vi "Inbetriebnahme_Marc.vi"() -> ()   [LabVIEW 2016]
panel:
  in  "Wicklungszahl n2 theoretisch":dbl=700.0
  out "Neukurve":cluster{"Y":dbl[], "Y":dbl[]}[](graph) caption="XY-Graph"
  in  "lm [cm]":dbl=94.0
  in  "Querschnitt A":dbl=45.0
  in  "Faktor Runge Kutta":dbl=700.0
  in  "Wicklungszahl n1 theoretisch":dbl=700.0
  in  "ShuntWiderstand [Ohm]":dbl=1.0
  in  "maximale Spannung":dbl=10.0
  in  "Messpunkte Oszi (6000)":i32=6000
  in  "VISA Name OZ in(OZ)":refnum<visa-resource-name>="USB0::0x0957::0x179B::MY54313507::INSTR"
  out "error out":errorcluster
  in  "Frequenz [Hz]":dbl
  in  "Spannungs Abweichung":dbl
  in  "Error_in":errorcluster
  in  "VISA Name FG in(FG)":refnum<visa-resource-name>="USB0::0x0957::0x0407::MY44043889::INSTR"
  # "Parameter Frequenzgenerator und Oszi"
  # "Parameter Messuaufbau"
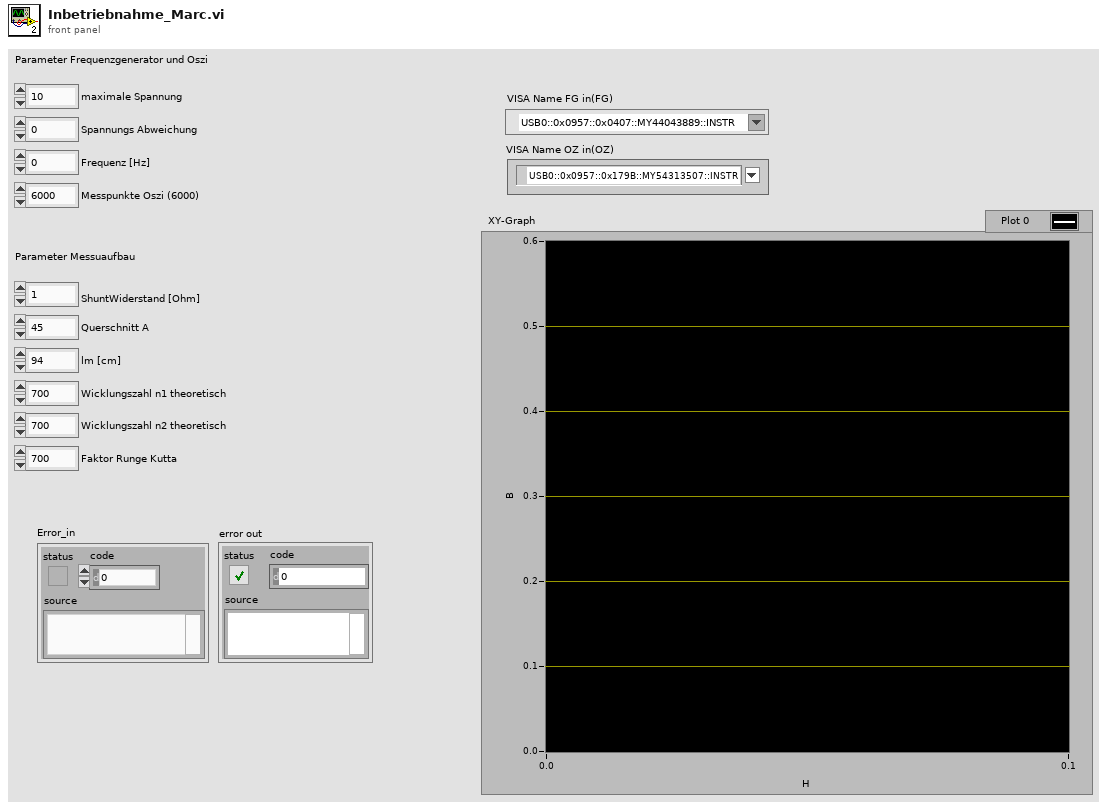
[diagram p1: front panel]
types:
  T1 = enum16{"Default", "FG Init", "Entmagnetisieren", "Oszi Init", "Messung Neukurve", "Plotten", "Ende"}
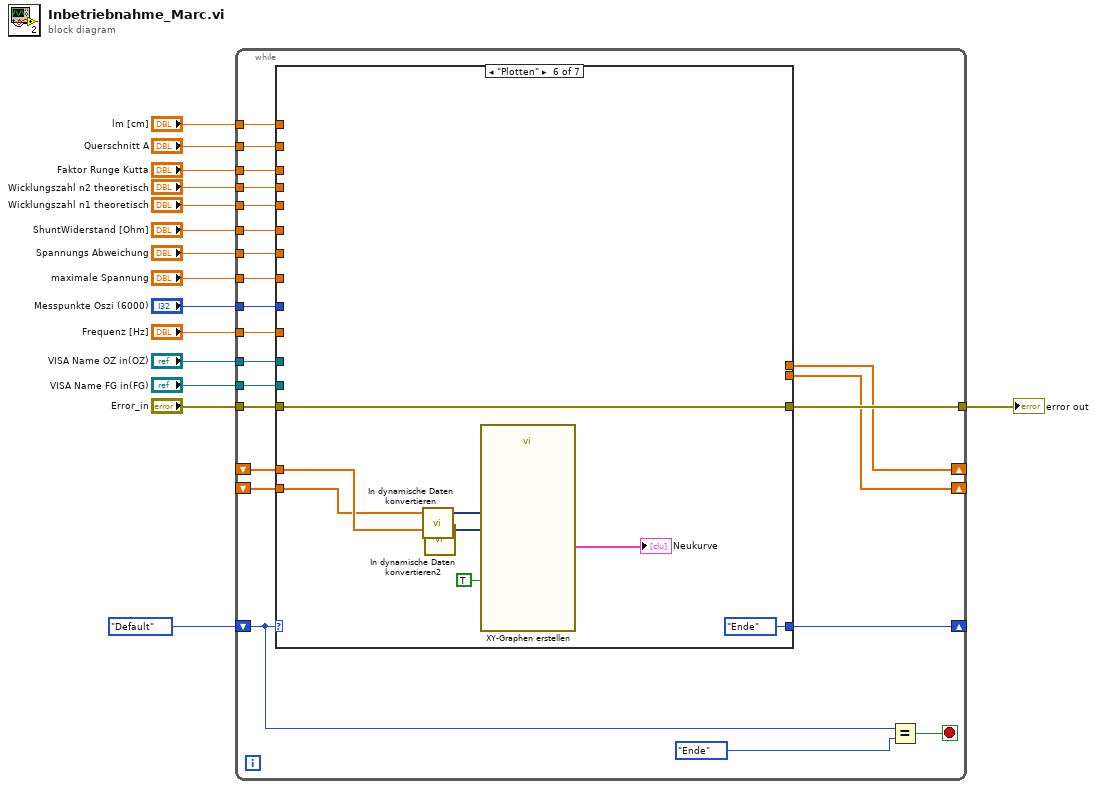
[diagram p0: block diagram]
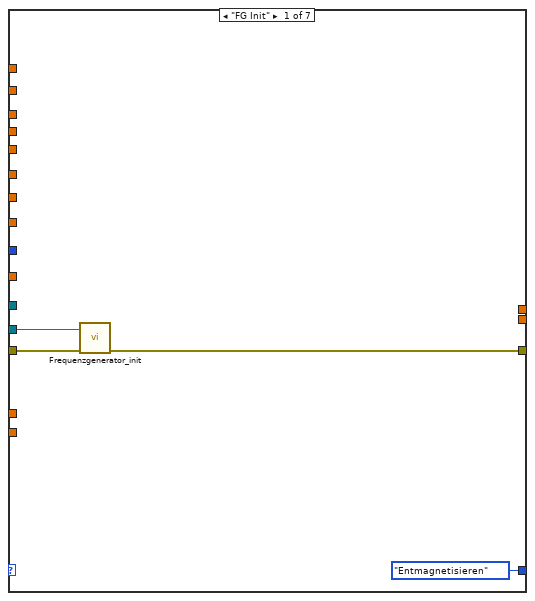
[diagram p2: hidden frame]
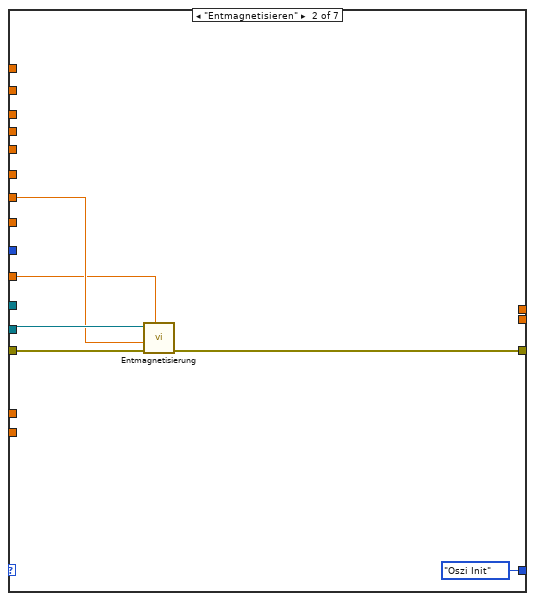
[diagram p3: hidden frame]
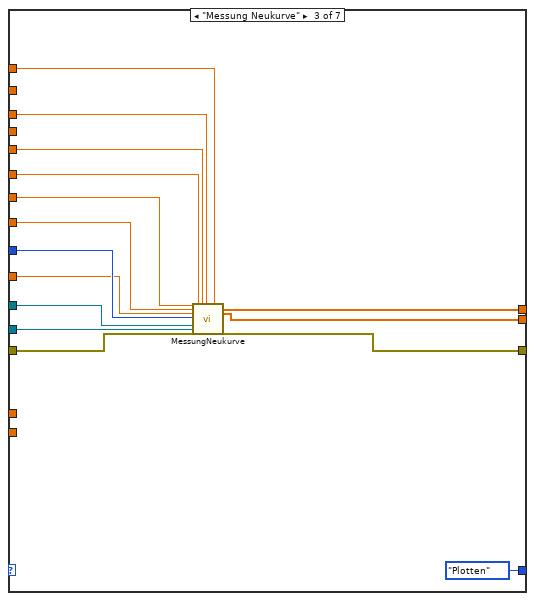
[diagram p4: hidden frame]
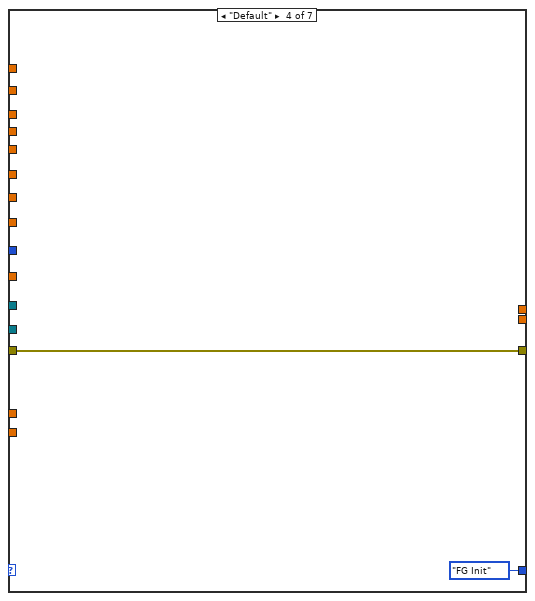
[diagram p5: hidden frame]
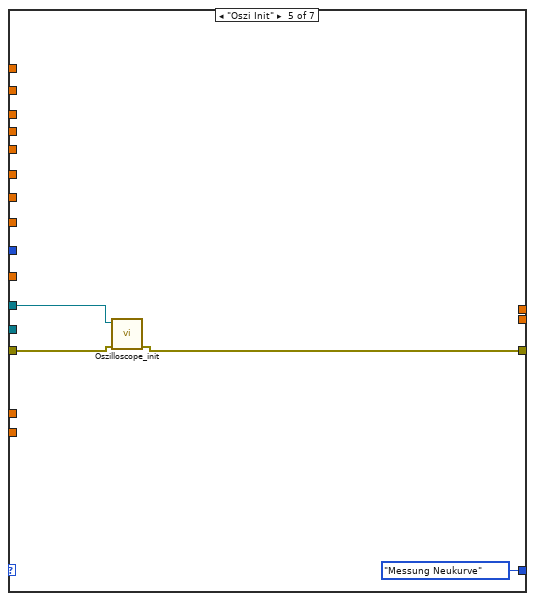
[diagram p6: hidden frame]
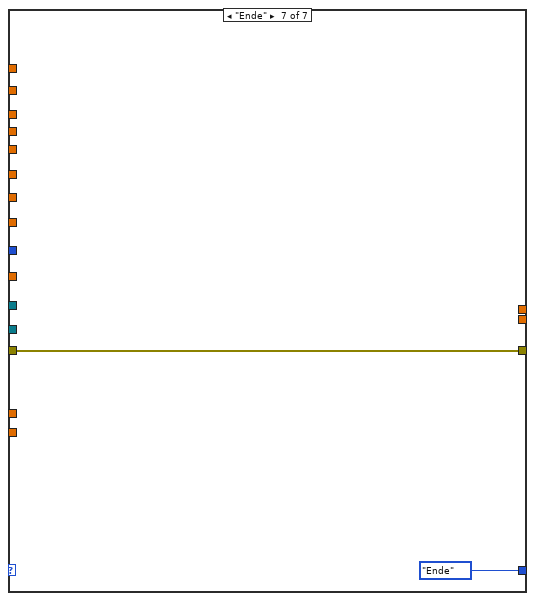
[diagram p7: hidden frame]
diagram:
  n1 = while {
    shift-right: [w35] -> _
    shift-left: T1."Default" -> [w32]
    tunnel: "VISA Name FG in(FG)" -> [w37]
    tunnel: "Error_in" -> [w36]
    tunnel: "Spannungs Abweichung" -> [w31]
    tunnel: "Frequenz [Hz]" -> [w30]
    tunnel: [w29] -> w10
    tunnel: "VISA Name OZ in(OZ)" -> [w28]
    tunnel: "Messpunkte Oszi (6000)" -> [w27]
    tunnel: "maximale Spannung" -> [w26]
    tunnel: "ShuntWiderstand [Ohm]" -> [w25]
    tunnel: "Wicklungszahl n1 theoretisch" -> [w24]
    tunnel: "Faktor Runge Kutta" -> [w23]
    tunnel: "Querschnitt A" -> [w22]
    tunnel: "lm [cm]" -> [w21]
    shift-right: [w20] -> _
    shift-left: _ -> [w18]
    shift-right: [w19] -> _
    shift-left: _ -> [w17]
    tunnel: "Wicklungszahl n2 theoretisch" -> [w16]
    stop <- w34 stop-if-true
    n2 = case shown="\"Plotten\"" w32 {
      tunnel: w37 -> [w41 w46 w60 _ _ _ _]
      tunnel: w36 -> [w40 w47 w62 w63 w68 w75 w77]
      tunnel: [T1."Entmagnetisieren" T1."Oszi Init" T1."Plotten" T1."FG Init" T1."Messung Neukurve" T1."Ende" T1."Ende"] -> w35
      tunnel: w31 -> [_ w45 w48 _ _ _ _]
      tunnel: w30 -> [_ w44 w57 _ _ _ _]
      tunnel: [w38 w43 w61 w63 w67 w75 w77] -> w29
      tunnel: w28 -> [_ _ w59 _ w66 _ _]
      tunnel: w27 -> [_ _ w58 _ _ _ _]
      tunnel: w26 -> [_ _ w56 _ _ _ _]
      tunnel: w25 -> [_ _ w55 _ _ _ _]
      tunnel: w24 -> [_ _ w54 _ _ _ _]
      tunnel: w23 -> [_ _ w53 _ _ _ _]
      tunnel: w22 -> [_ _ _ _ _ _ _]
      tunnel: w21 -> [_ _ w52 _ _ _ _]
      tunnel: [_ _ w50 _ _ _ _] -> w20
      tunnel: [_ _ w49 _ _ _ _] -> w19
      tunnel: w18 -> [_ _ _ _ _ w70 _]
      tunnel: w17 -> [_ _ _ _ _ w69 _]
      tunnel: w16 -> [_ _ _ _ _ _ _]
      frame "FG Init" {
        n3 = call "Frequenzgenerator_init.vi"("Error_in"=w40, "VISA Name FG in(FG)"=w41) -> ("Error_out"=w38:errorcluster)  [unwired: 8 in, 1 out]
      }
      frame "Entmagnetisieren" {
        n4 = call "Entmagnetisierung.vi"("Frequenz"=w44, "error in (no error)"=w47, "Spannungs Abweichung"=w45, "VISA Name FG in"=w46) -> ("error out"=w43:errorcluster)  [unwired: 6 in, 1 out]
      }
      frame "Messung Neukurve" {
        n5 = call "MessungNeukurve.vi"("Spannungs Abweichung"=w48, "maximale Spannung"=w56, "Frequency (1000 Hz)"=w57, "Messpunkte Oszi (6000)"=w58, "VISA Name OZ In (OZ)"=w59, "VISA Name FG in"=w60, "error in (no error)"=w62, "ShuntWiderstand [Ohm]"=w55, "Wicklungszahl n1 theoretisch"=w54, "Faktor Runge Kutta"=w53, "lm [cm]"=w52) -> ("Output B Array"=w50:dbl[], "Output H Array"=w49:dbl[], "error out"=w61:errorcluster)  [unwired: 11 in, 3 out]
      }
      frame "Default" {
      }
      frame "Oszi Init" {
        n6 = call "Oszilloscope_init.vi"("Error_in"=w68, "VISA Name OZ in(OZ)"=w66) -> ("Error_out"=w67:errorcluster)  [unwired: 8 in, 1 out]
      }
      frame "Plotten" {
        n7 = call "In dynamische Daten konvertieren"("Array"=w69) -> ("Dynamic Data Type"=w74:dynamicdata)  [unwired: 3 in]
        n8 = call "In dynamische Daten konvertieren2"("Array"=w70) -> ("Dynamic Data Type"=w73:dynamicdata)  [unwired: 3 in]
        n9 = call "XY-Graphen erstellen"("Enable"=TRUE, "Y Input"=w73, "X Input"=w74) -> ("XY Graph"=→"Neukurve":cluster{"X":dbl[], "Y":dbl[]}[])  [unwired: 7 in, 1 out]
      }
      frame "Ende" {
      }
    }
    n10 = Equal?(x=w32, y=T1."Ende") -> (x = y?=w34:bool)
  }
  "error out" <- w10
